vi "VI UUT_Complex.vi"(11 "Cluster control":T1) -> (3 "Cluster Indicator":T1)   [LabVIEW 2020, in "Test Scripting API.lvclass"]
uses:
  Test Scripting API.lvclass
  Test Scripting API.lvclass/Test Scripting API.ctl
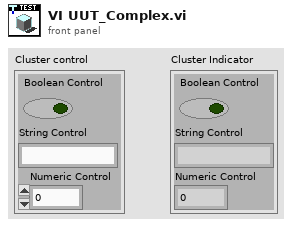
[diagram p1: front panel]
types:
  T1 = cluster{"Boolean Control":bool, "String Control":string, "Numeric Control":dbl}
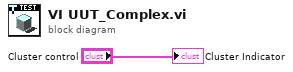
[diagram p0: block diagram]
diagram:
  "Cluster Indicator" <- "Cluster control"
